vi "[SubVI]Torque_Gage.vi"(2 "Left Offset":dbl, 3 "Right Offset":dbl, 4 "Left Input":dbl, 5 "Right Input":dbl) -> (0 "Right Torque":dbl, 1 "Left Torque":dbl)   [LabVIEW 2019]
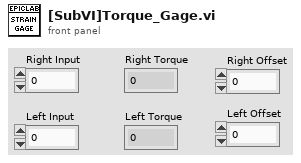
[diagram p1: front panel]
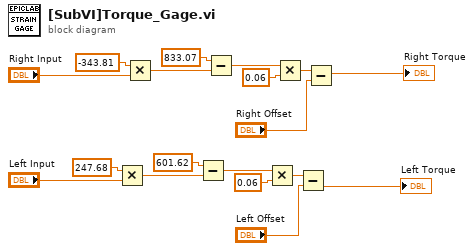
[diagram p0: block diagram]
diagram:
  n1 = Multiply(x=247.68, y="Left Input") -> (x*y=w11:dbl)
  n2 = Multiply(x=-343.81, y="Right Input") -> (x*y=w16:dbl)
  n3 = Subtract(x=601.62, y=w11) -> (x-y=w9:dbl)
  n4 = Subtract(x=833.07, y=w16) -> (x-y=w3:dbl)
  n5 = Multiply(x=w9, y=0.06) -> (x*y=w7:dbl)
  n6 = Multiply(x=w3, y=0.06) -> (x*y=w8:dbl)
  n7 = Subtract(x=w7, y="Left Offset") -> (x-y=→"Left Torque":dbl)
  n8 = Subtract(x=w8, y="Right Offset") -> (x-y=→"Right Torque":dbl)
